vi "Chroma 1905x Series 488.2 Cmd -ESE.vi"(8 "error in (no error)":errorcluster, 10 "decimal":i16 min=0 max=255 step=1, 11 "VISA resource name":refnum<visa-resource-name>) -> (0 "error out":errorcluster, 3 "VISA resource name out":refnum<visa-resource-name>)   [LabVIEW 2025]
panel:
  # "*ESE"
  # "Event Status Enable"
  # "0...255"
  # "Bit  Description\n0    Operation Complete\n1    Not Used\n2    Query Error\n3    Device Error\n4    Execution Error\n5    Command Error\n6    Not Used\n7    Power On"
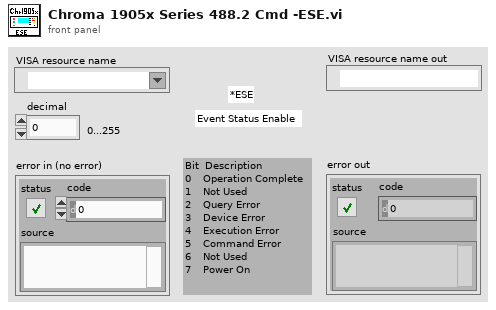
[diagram p1: front panel]
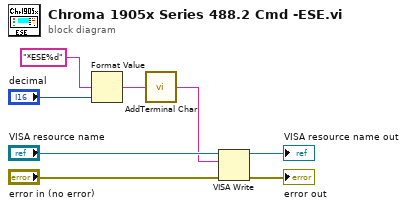
[diagram p0: block diagram]
diagram:
  n1 = Format Value(format string="*ESE%d", value (0)="decimal") -> (output string=w7:string)  [unwired: 1 in]
  n2 = call "AddTerminal Char.vi"("Cmd string"=w7) -> ("Concatenated String"=w1:string)  [unwired: 4 in]
  n3 = VISA Write(VISA resource name="VISA resource name", write buffer=w1, error in (no error)="error in (no error)") -> (VISA resource name out=→"VISA resource name out":refnum<visa-resource-name>, error out=→"error out":errorcluster)  [unwired: 1 out]
